vi "Write to UDP.vi"(8 "error in":errorcluster, 11 "Control Loop Cluster":T1) -> (0 "error out":errorcluster, 3 "Control Loop Cluster Out":T1)   [LabVIEW 2023, in "RT Main.lvlib"]
uses:
  RT Main.lvlib
  Control Loop Cluster.ctl
  <vilib>/myRIO/Instrument Drivers/Onboard IO/AI/typedefs/AI Reference.ctl
  <vilib>/myRIO/Common/Instrument Driver Framework/Utilities/typedefs/myRIO Generic Hardware Reference.ctl
  <vilib>/myRIO/Common/Instrument Driver Framework/Utilities/typedefs/Hardware Version Enum.ctl
  <vilib>/myRIO/Common/Instrument Driver Framework/Utilities/typedefs/myRIO v1.0 Reference.ctl
  <vilib>/myRIO/Common/Instrument Driver Framework/Utilities/typedefs/Generic FPGA Reference.ctl
  <vilib>/myRIO/Common/Instrument Driver Framework/myRIO v1.0/AI/typedefs/AI Channels List.ctl
  <vilib>/myRIO/Common/Instrument Driver Framework/myRIO v1.0/AI/typedefs/AI Channels Enum.ctl
  <vilib>/myRIO/Common/Instrument Driver Framework/Utilities/typedefs/Analog Scaling Constants List.ctl
  <vilib>/myRIO/Common/Instrument Driver Framework/Utilities/typedefs/Analog Scaling Constants.ctl
  <vilib>/myRIO/Instrument Drivers/Onboard IO/DIO/typedefs/DIO Reference.ctl
  <vilib>/myRIO/Common/Instrument Driver Framework/myRIO v1.0/DIO/typedefs/DIO Channels List.ctl
  <vilib>/myRIO/Common/Instrument Driver Framework/myRIO v1.0/DIO/typedefs/DIO Channels Enum.ctl
  Data Cluster.ctl
  Hardware Monitoring.ctl
  <vilib>/myRIO/Instrument Drivers/Onboard IO/AI/AI.lvlib
  <vilib>/myRIO/Instrument Drivers/Onboard IO/DIO/DIO.lvlib
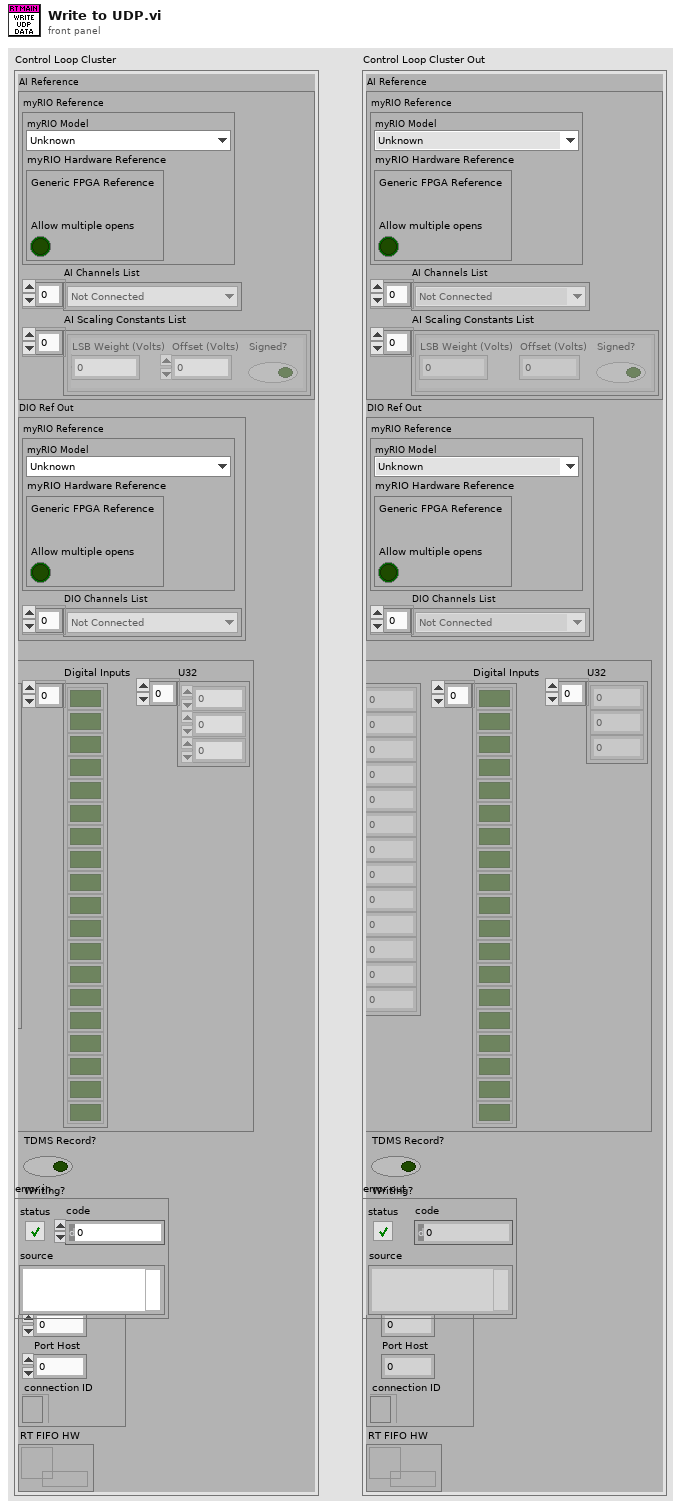
[diagram p1: front panel]
types:
  T1 = typedef "RT Main.lvlib/Control Loop Cluster.ctl" = cluster{"AI Reference":T2, "DIO Reference":T11, "Data Cluster":T14, "TDMS Record?":bool, "Writing?":bool, "UDP Info":cluster{"IP Host":string, "Port RT":u16, "Port Host":u16, "connection ID":refnum<k16>}, "RT FIFO HW":refnum<k33>}
  T2 = typedef "AI.lvlib/AI Reference.ctl" = cluster{"myRIO Reference":T3, "AI Channels List":T7, "AI Scaling Constants List":T9}
  T3 = typedef "myRIO Generic Hardware Reference.ctl" = cluster{"myRIO Model":T4, "myRIO Hardware Reference":T5}
  T4 = typedef "Hardware Version Enum.ctl" = enum16{"Unknown", "myRIO-1900", "myRIO-1950", "roboRIO", "NI ELVIS RIO CM", "ELVIS III"}
  T5 = typedef "myRIO v1.0 Reference.ctl" = cluster{"Generic FPGA Reference":T6, "Allow multiple opens":bool}
  T6 = typedef "Generic FPGA Reference.ctl" = refnum<k20>
  T7 = typedef "AI Channels List.ctl" = T8[]
  T8 = typedef "AI Channels Enum.ctl" = enum16{"Not Connected", "AudioIn/Left", "AudioIn/Right", "C/AI0", "C/AI1", "A/AI0", "A/AI1", "A/AI2", "A/AI3", "A/AI4", "A/AI5", "A/AI6", "A/AI7", "B/AI0", "B/AI1", "B/AI2", "B/AI3", "B/AI4", "B/AI5", "B/AI6", "B/AI7", "AI/AI0", "AI/AI1", "AI/AI2", "AI/AI3", "A/AI0 (DIFF)", "A/AI1 (DIFF)", "A/AI2 (DIFF)", "A/AI3 (DIFF)", "B/AI0 (DIFF)", "B/AI1 (DIFF)", "B/AI2 (DIFF)", "B/AI3 (DIFF)"}
  T9 = typedef "Analog Scaling Constants List.ctl" = T10[]
  T10 = typedef "Analog Scaling Constants.ctl" = cluster{"LSB Weight (Volts)":dbl, "Offset (Volts)":dbl, "Signed?":bool}
  T11 = typedef "DIO.lvlib/DIO Reference.ctl" = cluster{"myRIO Reference":T3, "DIO Channels List":T12}
  T12 = typedef "DIO Channels List.ctl" = T13[]
  T13 = typedef "DIO Channels Enum.ctl" = enum16{"Not Connected", "C/DIO0", "C/DIO1", "C/DIO2", "C/DIO3", "C/DIO4", "C/DIO5", "C/DIO6", "C/DIO7", "A/DIO0", "A/DIO1", "A/DIO2", "A/DIO3", "A/DIO4", "A/DIO5", "A/DIO6", "A/DIO7", "A/DIO8", "A/DIO9", "A/DIO10", "A/DIO11", "A/DIO12", "A/DIO13", "A/DIO14", "A/DIO15", "A/DIO16", "A/DIO17", "A/DIO18", "A/DIO19", "B/DIO0", "B/DIO1", "B/DIO2", "B/DIO3", "B/DIO4", "B/DIO5", "B/DIO6", "B/DIO7", "B/DIO8", "B/DIO9", "B/DIO10", "B/DIO11", "B/DIO12", "B/DIO13", "B/DIO14", "B/DIO15", "B/DIO16", "B/DIO17", "B/DIO18", "B/DIO19", "LED0", "LED1", "LED2", "LED3", "Button0", "DIO/DIO0", "DIO/DIO1", "DIO/DIO2", "DIO/DIO3", "DIO/DIO4", "DIO/DIO5", "DIO/DIO6", "DIO/DIO7", "DIO/DIO8", "DIO/DIO9", "SPI/CS0", "SPI/CS1", "SPI/CS2", "SPI/CS3", "LED RADIO (Green)", "LED RADIO (Red)", "LED COMM (Green)", "LED COMM (Red)", "LED MODE (Green)", "LED MODE (Red)"}
  T14 = typedef "RT Main.lvlib/Data Cluster.ctl" = cluster{"Analog Input":dbl[], "Digital Inputs":bool[], "U32":u32[]}
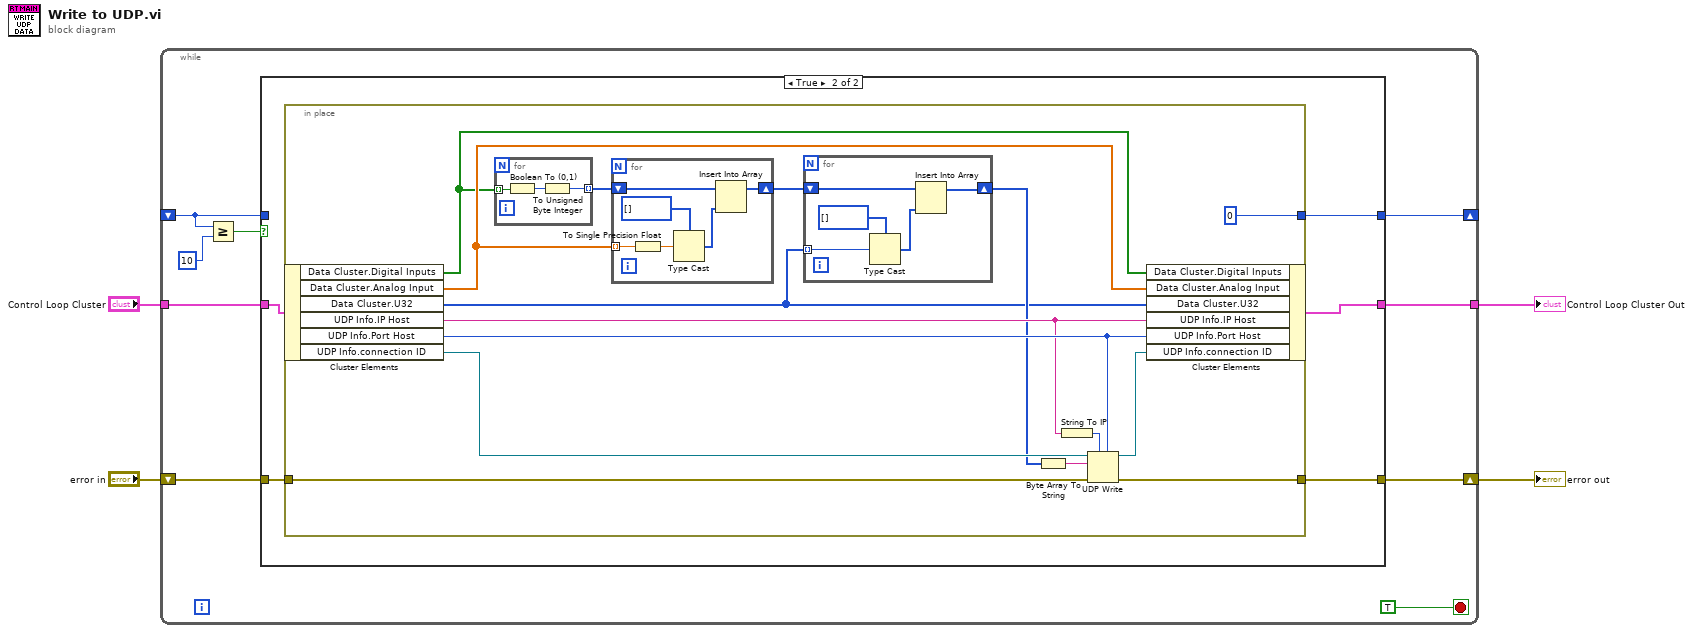
[diagram p0: block diagram]
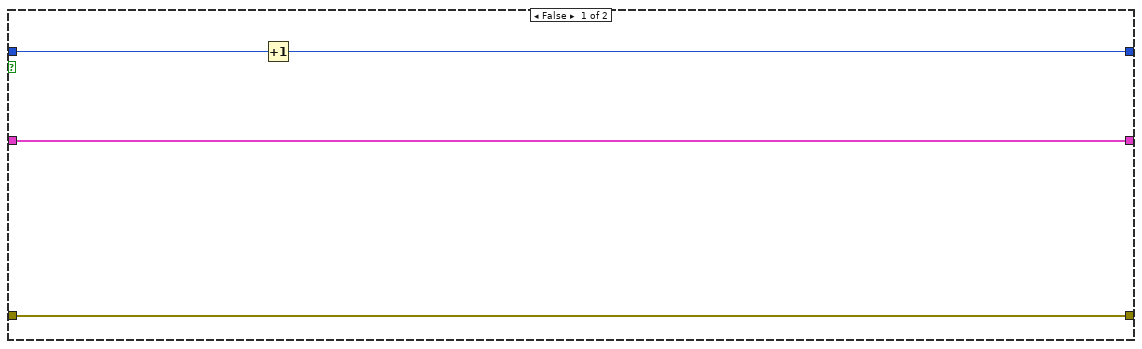
[diagram p2: hidden frame]
diagram:
  n1 = while {
    tunnel: "Control Loop Cluster" -> [w13]
    tunnel: [w11] -> w2
    shift-right: [w10] -> w1
    shift-left: "error in" -> [w12]
    shift-right: [w7] -> _
    shift-left: _ -> [w5]
    stop <- TRUE stop-if-true
    n2 = Greater Or Equal?(x=w5, y=10) -> (x >= y?=w8:bool)
    n3 = case shown="True" w8 {
      tunnel: w13 -> [w16 w22]
      tunnel: w12 -> [w17 w21]
      tunnel: [w16 w20] -> w11
      tunnel: [w17 w19] -> w10
      tunnel: [w14 w18] -> w7
      tunnel: w5 -> [w15 _]
      frame False {
        n4 = Increment(x=w15) -> (x+1=w14:i32)
      }
      frame True {
        n5 = in-place {
          in-place-border: w21 -> [w34]
          in-place-border: [w33] -> w19
          in-place-border: [0] -> w18
          n6 = in-place-cluster #1(w22) -> ("Data Cluster.Digital Inputs"=w35:bool[], "Data Cluster.Analog Input"=w36:dbl[], "Data Cluster.U32"=w23:u32[], "UDP Info.IP Host"=w28:string, "UDP Info.Port Host"=w31:u16, "UDP Info.connection ID"=w32:refnum<k16>)
          n7 = for {
            tunnel: w35 -> [w51] mode=indexing
            tunnel: [w49] -> w37 mode=indexing
            n8 = Boolean To (0,1)(Boolean=w51) -> (0, 1=w50:i16)
            n9 = To Unsigned Byte Integer(number=w50) -> (unsigned 8bit integer=w49:u8)
          }
          n10 = for {
            tunnel: w36 -> [w48] mode=indexing
            shift-right: [w44] -> w25
            shift-left: w37 -> [w43]
            n11 = To Single Precision Float(number=w48) -> (single precision float=w47:sgl)
            n12 = Type Cast(type=u8[] [], x=w47) -> (*(type *) &x=w45:u8[])
            n13 = Insert Into Array(array=w43, new element=w45) -> (w44:u8[])  [unwired: 1 in]
          }
          n14 = for {
            shift-right: [w38] -> w24
            shift-left: w25 -> [w40]
            tunnel: w23 -> [w42] mode=indexing
            n15 = Type Cast(type=u8[] [], x=w42) -> (*(type *) &x=w39:u8[])
            n16 = Insert Into Array(array=w40, new element=w39) -> (w38:u8[])  [unwired: 1 in]
          }
          n17 = Byte Array To String(unsigned byte array=w24) -> (string=w27:string)
          n18 = String To IP(1:w28) -> (0:w29:u32)
          n19 = UDP Write(address=w29, port or service name=w31, connection ID=w32, data in=w27, 8:w34) -> (error out=w33:errorcluster, 3:w30:refnum<k16>)  [unwired: 1 in]
          n20 = in-place-cluster #1("Data Cluster.Digital Inputs"=w35, "Data Cluster.Analog Input"=w36, "Data Cluster.U32"=w23, "UDP Info.IP Host"=w28, "UDP Info.Port Host"=w31, "UDP Info.connection ID"=w30) -> (w20:T1)
        }
      }
    }
  }
  "Control Loop Cluster Out" <- w2
  "error out" <- w1
